vi "Listen.vi"(8 "error in (no error)":errorcluster, 11 "Connection.Collection":refnum<class "Connection.Collection.lvclass">) -> (0 "error out":errorcluster, 3 "Connection.Collection":refnum<class "Connection.Collection.lvclass">)   [LabVIEW 2013, in "Connection_GOSPL.lvlib" / "Connection.Collection.lvclass"]
uses:
  Connection.Collection.lvclass
  Connection.Collection.lvclass/Connection.Collection.ctl
  map.ctl
  Connection/Connection.lvclass
  incoming connection.ctl
  wait_for_connection_process.vi
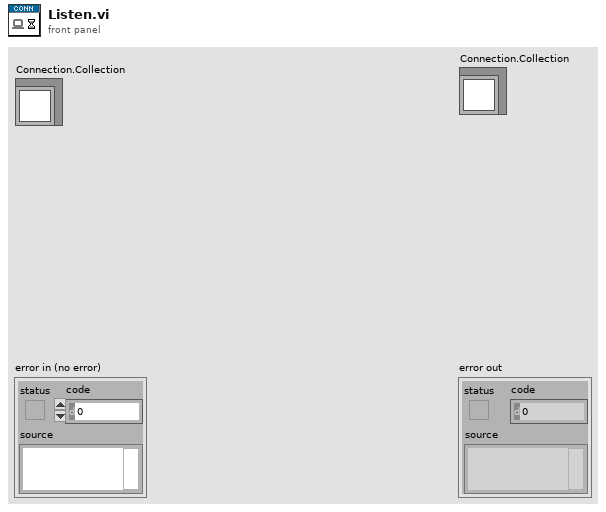
[diagram p1: front panel]
types:
  T1 = typedef "Connection_GOSPL.lvlib/Connection.Collection.lvclass/map.ctl" = cluster{"Connection":refnum<class "Connection.lvclass">, "Queue":refnum<queue>}
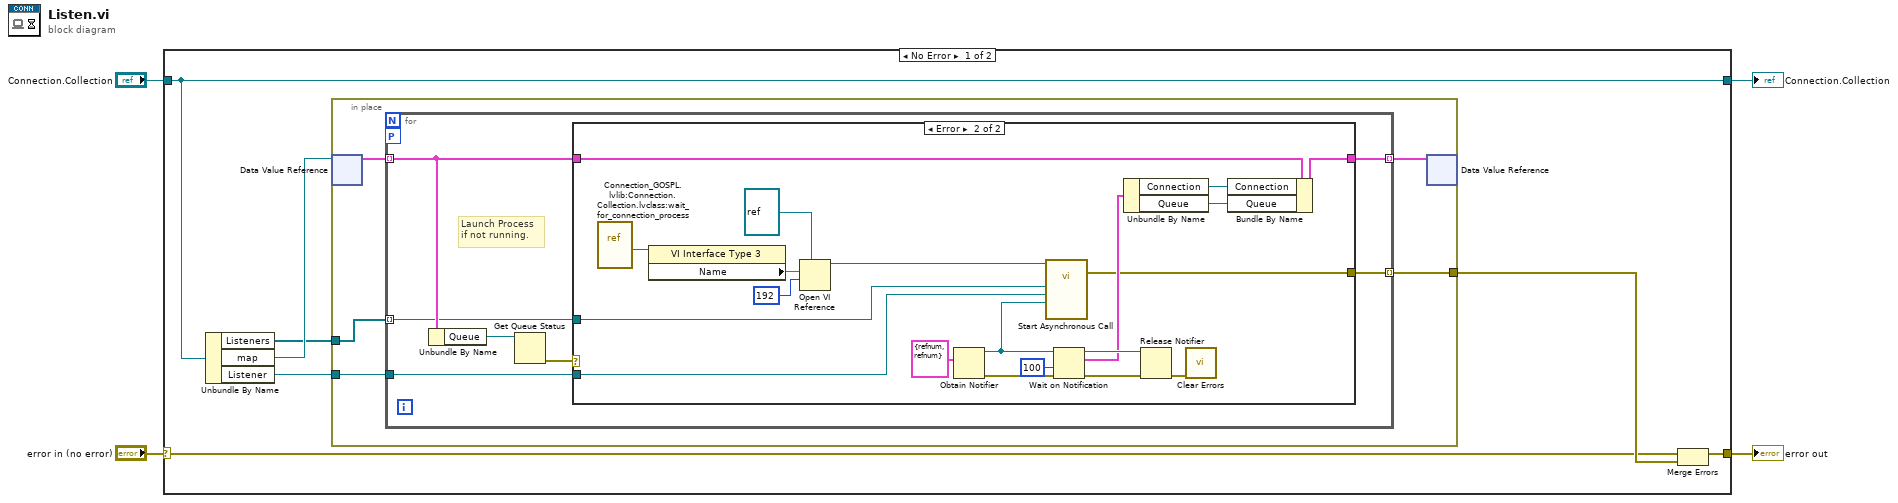
[diagram p0: block diagram]
diagram:
  n1 = case shown="No Error" "error in (no error)" {
    selector: "error in (no error)" -> [w9 w46]
    tunnel: [w11 w46] -> w3
    tunnel: [w8 w45] -> w2
    tunnel: "Connection.Collection" -> [w8 w45]
    frame No Error {
      n2 = Unbundle By Name(w8) -> ("Listeners"=w5:refnum<class "Connection.lvclass">[], "map"=w6:refnum<data-value>, "Listener"=w7:refnum<queue>)
      n3 = in-place {
        in-place-border: [w16] -> w10
        in-place-border: w7 -> [w15]
        in-place-border: w5 -> [w12]
        n4 = in-place-dvr #1(w6) -> (w14:T1[])  [unwired: 1 out]
        n5 = for {
          tunnel: [w23] -> w16 mode=indexing
          tunnel: w15 -> [w20]
          tunnel: w14 -> [w19] mode=indexing
          tunnel: [w18] -> w13 mode=indexing
          tunnel: w12 -> [w17] mode=indexing
          workers-P: _ -> [_]
          # "Launch Process\nif not running."
          n6 = Unbundle By Name(w19) -> ("Queue"=w21:refnum<queue>)
          n7 = Get Queue Status(queue=w21) -> (error out=w22:errorcluster)  [unwired: 2 in, 7 out]
          n8 = case shown="Error" w22 {
            tunnel: [_ w26] -> w23
            tunnel: w17 -> [_ w29]
            tunnel: w20 -> [_ w28]
            tunnel: w19 -> [w24 w37]
            tunnel: [w24 w36] -> w18
            frame No Error {
              # "Async process already launched."
            }
            frame Error {
              n9 = vi-ref "Connection_GOSPL.lvlib:Connection.Collection.lvclass:wait_for_connection_process.vi"() -> (w44:refnum<vi>)
              n10 = property class="VI Interface Type 3"(reference=w44) -> ("Name"=w43:string)  [unwired: 1 in, 2 out]
              n11 = Open VI Reference(type specifier VI Refnum (for type only)=refnum<vi> refnum, vi path=w43, options=192) -> (vi reference=w30:refnum<vi>)  [unwired: 3 in, 1 out]
              n12 = Obtain Notifier(notification data type=T1 {"Connection"=refnum, "Queue"=refnum} ("notification")) -> (notifier out=w27:refnum<notifier>, error out=w33:errorcluster)  [unwired: 3 in, 1 out]
              n13 = call-by-ref "Start Asynchronous Call"(reference=w30, "Notifier"=w27, "Queue"=w28, "Connection"=w29) -> (error out=w26:errorcluster)  [unwired: 10 in, 1 out]
              n14 = Wait on Notification(notifier=w27, timeout in ms (-1)=100, error in (no error)=w33) -> (notifier out=w38:refnum<notifier>, notification=w35:T1, error out=w32:errorcluster)  [unwired: 1 in, 1 out]
              n15 = Unbundle By Name(w35) -> ("Connection"=w25:refnum<class "Connection.lvclass">, "Queue"=w34:refnum<queue>)
              n16 = Release Notifier(notifier=w38, error in (no error)=w32) -> (error out=w31:errorcluster)  [unwired: 1 in, 2 out]
              n17 = call <vilib>:"Clear Errors.vi"("error in (no error)"=w31) -> ()  [unwired: 6 in, 1 out]
              n18 = Bundle By Name(cluster=w37, "Connection"=w25, "Queue"=w34) -> (w36:T1)
            }
          }
        }
        n19 = in-place-dvr #1(w13) -> ()  [unwired: 2 out]
      }
      n20 = Merge Errors(w9, w10) -> (w11:errorcluster)
    }
    frame Error {
    }
  }
  "error out" <- w3
  "Connection.Collection" <- w2
